vi "RP calculate subset CMA.vi"(5 "Samples per trigger increment":i32=2, 6 "Round off":i32=1024 format="0x%x (%d)", 7 "RAM size":i32=268435456 format="0x%x (%d)", 8 "Trigger start position":i32 format="0x%x (%d)", 9 "Pre-trigger samples":i32=125000 format="0x%x (%d)", 10 "Bytes per sample":i32=4, 11 "Post-trigger samples":i32=50000000 format="0x%x (%d)") -> (0 "Merged subsets":u64[](array[numeric]) format="0x%x (%d)", 1 "record length":i32 format="0x%x (%d)", 2 "pre-trigger trim":i32 format="0x%x (%d)", 3 "Subsets":i32[][](array[numeric]) format="0x%x (%d)")   [LabVIEW 2024]
uses:
  Mode.ctl
panel:
  out "RAM locations":i32[][](array[numeric]) format="0x%x (%d)"
  out "end_pos":i32 format="0x%x (%d)"
  out "start_pos":i32 format="0x%x (%d)"
  out "actual trigger pos":i32 format="0x%x (%d)"
  out "unsigned 64bit integer":u64[](array[numeric]) format="%x"
  out "x << y":u64 format="%x"
  out "post-trigger trim":i32
  out "subset end":i32 format="0x%x (%d)"
  out "subset start":i32 format="0x%x (%d)"
  in  "Mode":T1=enum."Digitizer"
  # "ends"
  # "starts"
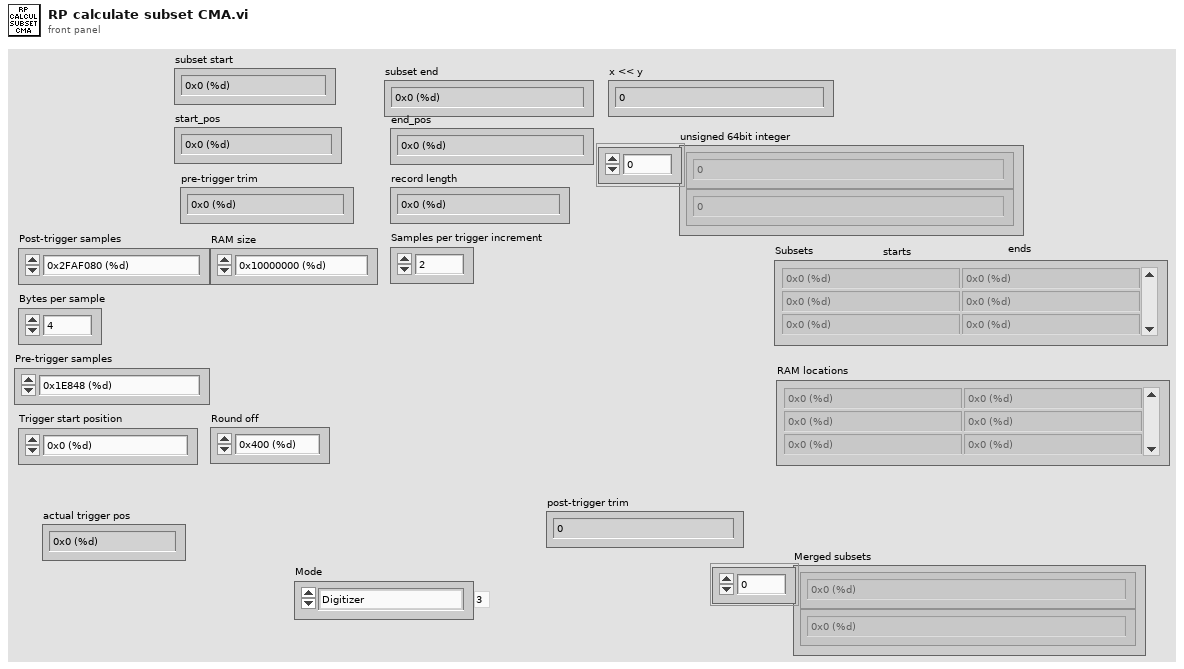
[diagram p1: front panel]
types:
  T1 = typedef "Mode.ctl" = enum16{"Filter", "Lockin test", "Snapshot test", "Digitizer", "Current-Voltage"}
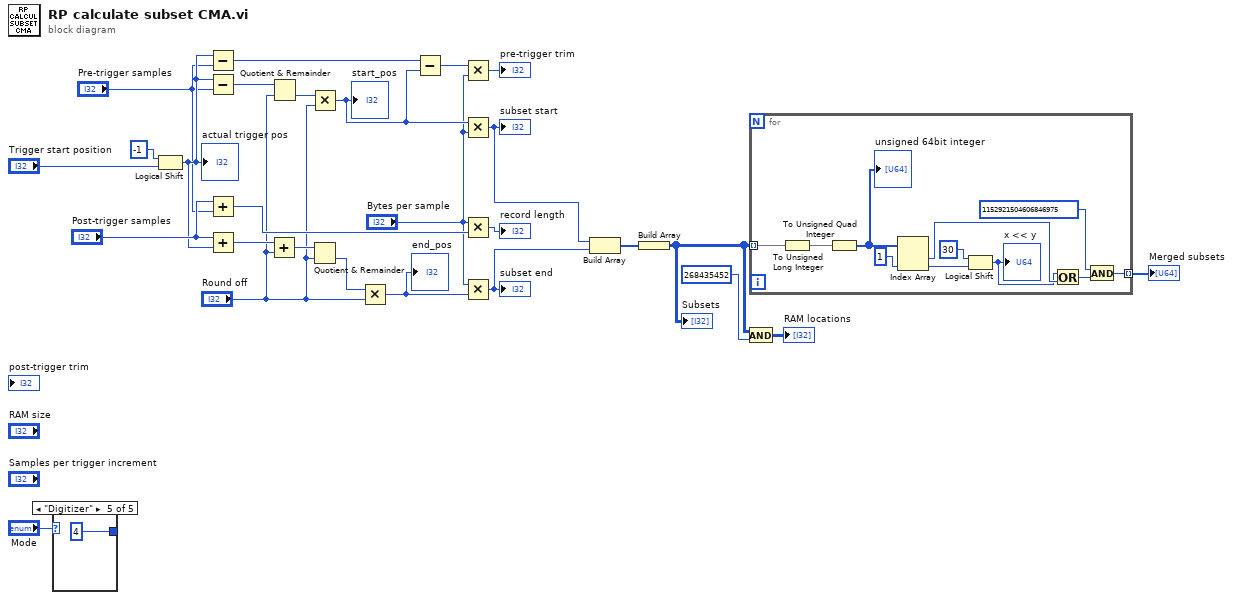
[diagram p0: block diagram]
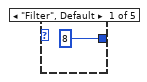
[diagram p2: hidden frame]
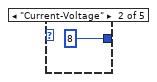
[diagram p3: hidden frame]
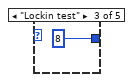
[diagram p4: hidden frame]
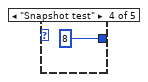
[diagram p5: hidden frame]
diagram:
  n1 = case shown="\"Digitizer\"" "Mode" {
    tunnel: [8 8 8 8 4] -> _
    frame "Filter", Default {
    }
    frame "Current-Voltage" {
    }
    frame "Lockin test" {
    }
    frame "Snapshot test" {
    }
    frame "Digitizer" {
    }
  }
  n2 = Logical Shift(y=i16 -1, x="Trigger start position") -> (x << y=w7:i32)
  "actual trigger pos" <- w7
  n3 = Subtract(x=w7, y="Pre-trigger samples") -> (x-y=w5:i32)
  n4 = Subtract(x=w7, y="Pre-trigger samples") -> (x-y=w17:i32)
  n5 = Add(x="Post-trigger samples", y="Pre-trigger samples") -> (x+y=w19:i32)
  n6 = Add(x="Post-trigger samples", y=w7) -> (x+y=w26:i32)
  n7 = Add(x=w26, y="Round off") -> (x+y=w13:i32)
  n8 = Quotient & Remainder(x=w17, y="Round off") -> (floor(x/y)=w25:i32)  [unwired: 1 out]
  n9 = Multiply(x=w25, y="Round off") -> (x*y=w4:i32)
  "start_pos" <- w4
  n10 = Quotient & Remainder(x=w13, y="Round off") -> (floor(x/y)=w24:i32)  [unwired: 1 out]
  n11 = Multiply(x=w24, y="Round off") -> (x*y=w20:i32)
  "end_pos" <- w20
  n12 = Subtract(x=w5, y=w4) -> (x-y=w3:i32)
  n13 = Multiply(x=w3, y="Bytes per sample") -> (x*y=→"pre-trigger trim":i32)
  n14 = Multiply(x=w4, y="Bytes per sample") -> (x*y=w16:i32)
  "subset start" <- w16
  n15 = Multiply(x="Bytes per sample", y=w19) -> (x*y=→"record length":i32)
  n16 = Multiply(x="Bytes per sample", y=w20) -> (x*y=w11:i32)
  "subset end" <- w11
  n17 = Build Array(w16, w11) -> (w23:i32[])
  n18 = Build Array(w23) -> (w10:i32[][])
  "Subsets" <- w10
  n19 = And(x=w10, y=268435452) -> (x .and. y?=→"RAM locations":i32[][])
  n20 = for {
    tunnel: w10 -> [w43] mode=indexing
    tunnel: [w35] -> w21 mode=indexing
    n21 = To Unsigned Long Integer(number=w43) -> (unsigned 32bit integer=w33:u32[])
    n22 = To Unsigned Quad Integer(1:w33) -> (0:w42:u64[])
    "unsigned 64bit integer" <- w42
    n23 = Index Array(array=w42, index #2=1 ("index")) -> (element #1=w38:u64, element #2=w40:u64)  [unwired: 1 in]
    n24 = Logical Shift(y=i16 30, x=w40) -> (x << y=w37:u64)
    "x << y" <- w37
    n25 = Or(x=w37, y=w38) -> (x .or. y?=w36:u64)
    n26 = And(x=u64 1152921504606846975 ("value"), y=w36) -> (x .and. y?=w35:u64)
  }
  "Merged subsets" <- w21
